vi "PongVIEW.vi"() -> ()   [LabVIEW 2015]
uses:
  Instance           1 18Saved   pong_state .vi
  user32.dll
panel:
  out "Paddle":dbl(slide) scale=0.0..1366.0
  out "Game Over String":string
  out "Paddle Value":dbl
  out "Ball On Paddle?":bool
  out "Y Hit Upper Boundary?":bool
  out "Y Hit Lower Boundary?":bool
  out "X Hit Upper Boundary?":bool
  out "X Hit Lower Boundary?":bool
  out "CursorX":i32
  out "Ball Y Velocity":dbl=5.0
  out "Ball Y Position":dbl
  out "Ball X Velocity":dbl
  out "Ball X Position":dbl
  out "Height":i16
  out "Width":i16
  in  "Start Button":bool
  in  "Stop Button":bool
  out "XY Graph":cluster{"Y":dbl[], "Y":dbl[]}[](graph)
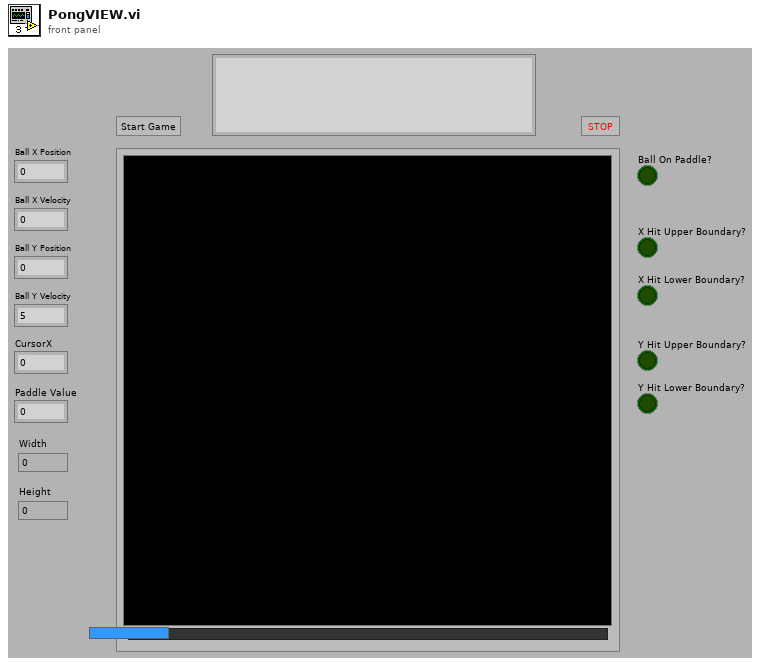
[diagram p1: front panel]
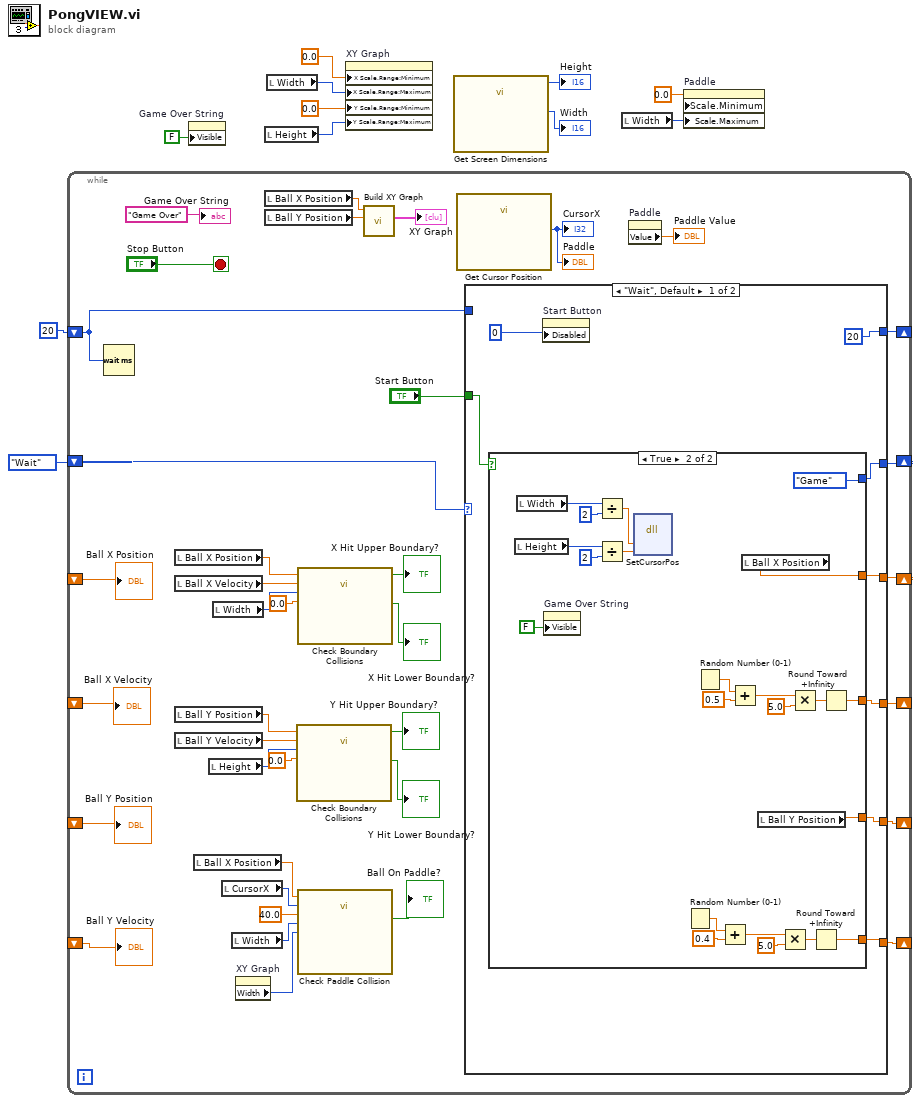
[diagram p0: block diagram]
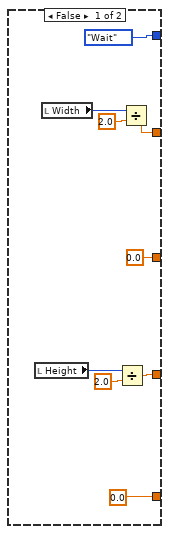
[diagram p2: hidden frame]
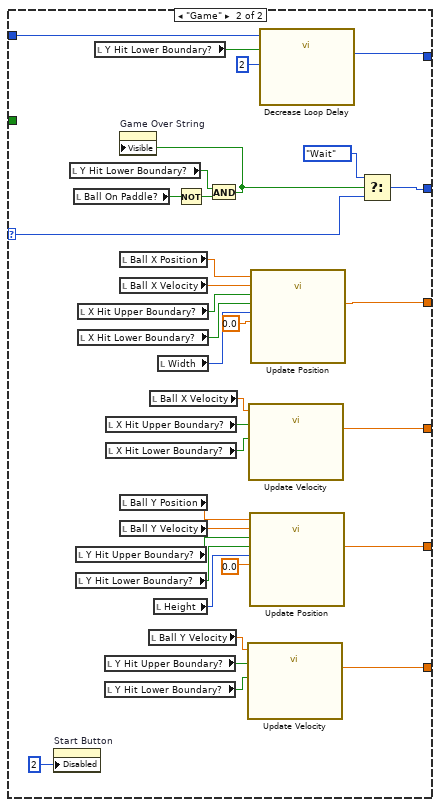
[diagram p3: hidden frame]
diagram:
  n1 = while {
    shift-right: [w45] -> _
    shift-left: _ -> [w41]
    shift-right: [w43] -> _
    shift-left: _ -> [w39]
    shift-right: [w44] -> _
    shift-left: _ -> [w40]
    shift-right: [w42] -> _
    shift-left: _ -> [w38]
    shift-right: [w48] -> _
    shift-left: enum16{"Wait", "Game"}."Wait" -> [w49]
    shift-right: [w22] -> _
    shift-left: u32 20 ("milliseconds to wait") -> [w23]
    stop <- "Stop Button" stop-if-true
    n2 = Wait (ms)(milliseconds to wait=w23) -> ()  [unwired: 1 out]
    n3 = local read "Ball X Position"() -> (w35:dbl)
    n4 = local read "Ball X Velocity"() -> (w34:dbl)
    n5 = local read "Ball Y Position"() -> (w33:dbl)
    n6 = local read "Ball Y Velocity"() -> (w32:dbl)
    n7 = local read "Ball X Position"() -> (w19:dbl)
    n8 = local read "Height"() -> (w25:i16)
    n9 = local read "Width"() -> (w29:i16)
    n10 = local read "CursorX"() -> (w18:i32)
    n11 = local read "Width"() -> (w20:i16)
    n12 = property on="XY Graph" class="XYGraph (strict)"() -> ("Width"=w13:u32)  [unwired: 2 in, 2 out]
    n13 = local read "Ball X Position"() -> (w37:dbl)
    n14 = local read "Ball Y Position"() -> (w36:dbl)
    n15 = call "Check Boundary Collisions.vi"("Lower Boundary"=0.0, "Upper Boundary"=w25, "Velocity"=w32, "Position"=w33) -> ("Hit Lower Boundary?"=→"Y Hit Lower Boundary?":bool, "Hit Upper Boundary?"=→"Y Hit Upper Boundary?":bool)  [unwired: 6 in]
    n16 = call "Check Boundary Collisions.vi"("Lower Boundary"=0.0 ("y"), "Upper Boundary"=w29, "Velocity"=w34, "Position"=w35) -> ("Hit Lower Boundary?"=→"X Hit Lower Boundary?":bool, "Hit Upper Boundary?"=→"X Hit Upper Boundary?":bool)  [unwired: 6 in]
    n17 = call "Check Paddle Collision.vi"("Screen Width"=w20, "Plot Width"=w13, "Paddle Radius"=40.0 ("y"), "CursorX"=w18, "Ball X Position"=w19) -> ("Ball On Paddle?"=→"Ball On Paddle?":bool)  [unwired: 6 in]
    n18 = call "Build XY Graph"("Y Input"=w36, "X Input"=w37) -> ("XY Graph"=→"XY Graph":cluster{"Y":dbl[], "Y":dbl[]}[])  [unwired: 8 in, 1 out]
    n19 = call "Get Cursor Position.vi"() -> ("CursorX"=→"CursorX" →"Paddle":i32)  [unwired: 10 in, 1 out]
    n20 = case shown="\"Wait\", Default" w49 {
      selector: w49 -> [_ w96]
      tunnel: [w54 w101] -> w43
      tunnel: [w53 w119] -> w45
      tunnel: [w56 w120] -> w44
      tunnel: [w55 w100] -> w42
      tunnel: [w52 w95] -> w48
      tunnel: "Start Button" -> [w51 _]
      tunnel: w23 -> [_ w94]
      tunnel: [u32 20 ("milliseconds to wait") w92] -> w22
      frame "Wait", Default {
        n21 = case shown="True" w51 {
          tunnel: [0.0 w84] -> w56
          tunnel: [0.0 w81] -> w55
          tunnel: [w60 w88] -> w54
          tunnel: [w59 w87] -> w53
          tunnel: [enum16{"Wait", "Game"}."Wait" enum16{"Wait", "Game"}."Game"] -> w52
          frame False {
            n22 = local read "Height"() -> (w63:i16)
            n23 = local read "Width"() -> (w64:i16)
            n24 = Divide(x=w63, y=2.0) -> (x/y=w60:dbl)
            n25 = Divide(x=w64, y=2.0) -> (x/y=w59:dbl)
          }
          frame True {
            n26 = local read "Height"() -> (w73:i16)
            n27 = local read "Width"() -> (w72:i16)
            n28 = property on="Game Over String" class="Str"("Visible"=FALSE) -> ()  [unwired: 2 in, 2 out]
            n29 = Divide(x=w72, y=2) -> (x/y=w71:dbl)
            n30 = Divide(x=w73, y=2) -> (x/y=w70:dbl)
            n31 = dll-call lib="user32.dll" fn="SetCursorPos"("X"=w71, "Y"=w70) -> ()  [unwired: 6 in, 2 out]
            n32 = Random Number (0-1)() -> (number: 0 to 1=w79:dbl)
            n33 = Random Number (0-1)() -> (number: 0 to 1=w69:dbl)
            n34 = Add(x=w79, y=0.4) -> (x+y=w77:dbl)
            n35 = Add(x=w69, y=0.5) -> (x+y=w67:dbl)
            n36 = local read "Ball X Position"() -> (w87:dbl)
            n37 = local read "Ball Y Position"() -> (w88:dbl)
            n38 = Multiply(x=w77, y=5.0) -> (x*y=w82:dbl)
            n39 = Multiply(x=w67, y=5.0) -> (x*y=w85:dbl)
            n40 = Round Toward +Infinity(x=w82) -> (ceil(x): smallest int >= x=w81:dbl)
            n41 = Round Toward +Infinity(x=w85) -> (ceil(x): smallest int >= x=w84:dbl)
          }
        }
        n42 = property on="Start Button" class="Bool"("Disabled"=u8 0) -> ()  [unwired: 2 in, 2 out]
      }
      frame "Game" {
        n43 = property on="Start Button" class="Bool"("Disabled"=u8 2) -> ()  [unwired: 2 in, 2 out]
        n44 = local read "Y Hit Lower Boundary?"() -> (w93:bool)
        n45 = local read "Ball On Paddle?"() -> (w99:bool)
        n46 = local read "Y Hit Upper Boundary?"() -> (w102:bool)
        n47 = local read "Y Hit Lower Boundary?"() -> (w103:bool)
        n48 = local read "X Hit Upper Boundary?"() -> (w114:bool)
        n49 = local read "X Hit Lower Boundary?"() -> (w113:bool)
        n50 = local read "Y Hit Lower Boundary?"() -> (w89:bool)
        n51 = local read "Y Hit Upper Boundary?"() -> (w106:bool)
        n52 = local read "Y Hit Lower Boundary?"() -> (w107:bool)
        n53 = local read "X Hit Upper Boundary?"() -> (w109:bool)
        n54 = local read "X Hit Lower Boundary?"() -> (w108:bool)
        n55 = local read "Ball X Position"() -> (w118:dbl)
        n56 = local read "Ball X Velocity"() -> (w117:dbl)
        n57 = local read "Ball Y Position"() -> (w112:dbl)
        n58 = local read "Ball Y Velocity"() -> (w111:dbl)
        n59 = local read "Ball Y Velocity"() -> (w110:dbl)
        n60 = local read "Ball X Velocity"() -> (w121:dbl)
        n61 = local read "Height"() -> (w104:i16)
        n62 = local read "Width"() -> (w115:i16)
        n63 = Not(x=w99) -> (.not. x?=w98:bool)
        n64 = And(x=w93, y=w98) -> (x .and. y?=w91:bool)
        n65 = property on="Game Over String" class="Str"("Visible"=w91) -> ()  [unwired: 2 in, 2 out]
        n66 = call "Update Velocity.vi"("Hit Lower Boundary?"=w107, "Hit Upper Boundary?"=w106, "Velocity"=w110) -> ("Updated Velocity"=w100:dbl)  [unwired: 8 in]
        n67 = call "Update Velocity.vi"("Hit Lower Boundary?"=w108, "Hit Upper Boundary?"=w109, "Velocity"=w121) -> ("Updated Velocity"=w120:dbl)  [unwired: 8 in]
        n68 = call "Update Position.vi"("Upper Boundary"=w104, "Lower Boundary"=0.0, "Hit Lower Boundary?"=w103, "Hit Upper Boundary?"=w102, "Velocity"=w111, "Position"=w112) -> ("Updated Position"=w101:dbl)  [unwired: 5 in]
        n69 = call "Update Position.vi"("Upper Boundary"=w115, "Lower Boundary"=0.0 ("t"), "Hit Lower Boundary?"=w113, "Hit Upper Boundary?"=w114, "Velocity"=w117, "Position"=w118) -> ("Updated Position"=w119:dbl)  [unwired: 5 in]
        n70 = call "Decrease Loop Delay.vi"("Amount to Decrease"=u32 2, "Y Hit Lower Boundary?"=w89, "Current Delay"=w94) -> ("Next Delay"=w92:u32)  [unwired: 8 in]
        n71 = Select(t=enum16{"Wait", "Game"}."Wait", s=w91, f=w96) -> (s? t:f=w95:enum16{"Wait", "Game"})
      }
    }
    n72 = property on="Paddle" class="Slide (strict)"() -> ("Value"=→"Paddle Value":dbl)  [unwired: 2 in, 2 out]
    "Ball X Position" <- w41
    "Ball X Velocity" <- w40
    "Ball Y Position" <- w39
    "Ball Y Velocity" <- w38
    "Game Over String" <- "Game Over" ("String")
  }
  n73 = property on="Game Over String" class="Str"("Visible"=FALSE) -> ()  [unwired: 2 in, 2 out]
  n74 = local read "Height"() -> (w8:i16)
  n75 = local read "Width"() -> (w7:i16)
  n76 = property on="XY Graph" class="XYGraph (strict)"("X Scale.Range:Minimum"=0.0, "X Scale.Range:Maximum"=w7, "Y Scale.Range:Minimum"=0.0, "Y Scale.Range:Maximum"=w8) -> ()  [unwired: 2 in, 2 out]
  n77 = call "Get Screen Dimensions.vi"() -> ("screenWidth"=→"Width":i32, "screenHeight"=→"Height":i32)  [unwired: 10 in]
  n78 = local read "Width"() -> (w1:i16)
  n79 = property on="Paddle" class="Slide (strict)"("Scale.Minimum"=0.0 ("Data Range:Minimum"), "Scale.Maximum"=w1) -> ()  [unwired: 2 in, 2 out]
